vi "Kill.vi"(7 "timeout [ms]":i32, 8 "error in":errorcluster, 11 "pipe in":T1) -> (0 "error out":errorcluster, 3 "pipe out":T1)   [LabVIEW 2020, in "LV Process library.lvlib"]
doc: "Calls lv_proc.dll to kill process. First asks operating system to end the process and waits. If timeout runs out the process is terminated. This VI is recommended to use only if there is no other way how to force process exit. If timeout is set to zero, vi waits indefinitely till the end of the process.\n\n---\nLV Process works only with lv_proc.dll library, which is part of vipm package or should be delivered together with packed library. Placement of this dll is selected in terminal of Create Process.vi."
uses:
  LV Process library.lvlib
  Pipe Handle.ctl
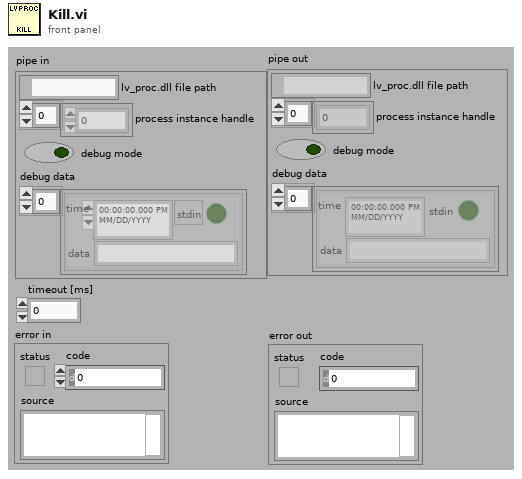
[diagram p1: front panel]
types:
  T1 = typedef "LV Process library.lvlib/Pipe Handle.ctl" = cluster{"lv_proc.dll file path":path, "process instance handle":u32[], "debug mode":bool, "debug data":cluster{"time":timestamp, "stdin":bool, "data":string}[]}
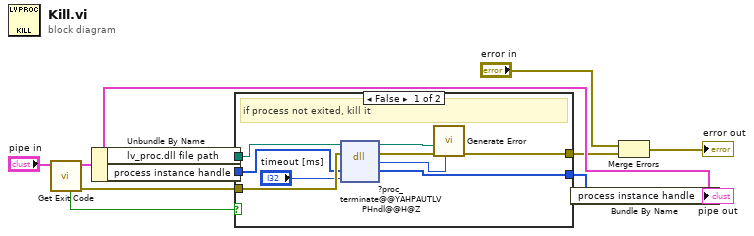
[diagram p0: block diagram]
diagram:
  n1 = call "Get Exit Code.vi"("pipe in"="pipe in") -> ("error out"=w5:errorcluster, "pipe out"=w7:T1, "exited?"=w1:bool)  [unwired: 6 in, 2 out]
  n2 = Unbundle By Name(w7) -> ("lv_proc.dll file path"=w11:path, "process instance handle"=w6:u32[])
  n3 = case shown="False" w1 {
    tunnel: [w13 w21] -> w4
    tunnel: w5 -> [w20 w21]
    tunnel: w6 -> [w19 w22]
    tunnel: [w12 w22] -> w9
    tunnel: w11 -> [w17 _]
    frame False {
      # "if process not exited, kill it"
      n4 = dll-call lib="C:/Data/GOLPI/LV Process/lv_proc.dll" fn="?proc_terminate@@YAHPAUTLVPHndl@@H@Z" label="proc_terminate"(path in=w17, error in=w20, "proc"=w19, "timeout [ms]"="timeout [ms]") -> (path out=w14:path, error out=w15:errorcluster, "error"=w16:i32, "proc"=w12:u32[])  [unwired: 2 in]
      n5 = call "Generate Error.vi"("error code in"=w16, "error in"=w15, "lv_proc.dll path in"=w14) -> ("error out"=w13:errorcluster)  [unwired: 6 in, 1 out]
    }
    frame True {
    }
  }
  n6 = Bundle By Name(cluster=w7, "process instance handle"=w9) -> (→"pipe out":T1)
  n7 = Merge Errors("error in", w4) -> (→"error out":errorcluster)
